vi "Update Status.vi"(8 "error in (no error)":errorcluster, 10 "Value":string, 11 "Status Ref":refnum<vi>) -> (0 "error out":errorcluster)   [LabVIEW 2025, in "I2C Bus Monitor UI.lvlib"]
uses:
  I2C Bus Monitor UI.lvlib
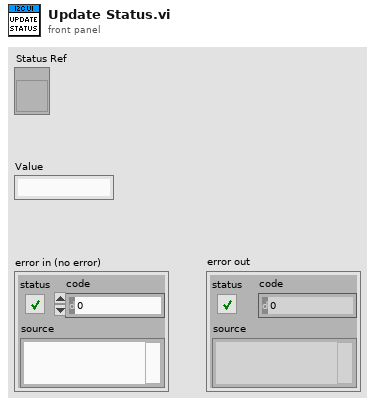
[diagram p1: front panel]
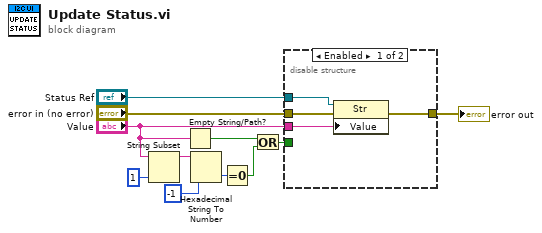
[diagram p0: block diagram]
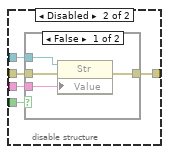
[diagram p2: hidden frame]
diagram:
  n1 = String Subset(string="Value", length (rest)=1 ("length (rest)")) -> (substring=w3:string)  [unwired: 1 in]
  n2 = Empty String/Path?(string/path="Value") -> (empty?=w6:bool)
  n3 = Hexadecimal String To Number(string=w3, default (0uL)=-1 ("default (0 U32)")) -> (number=w7:i32)  [unwired: 1 in, 1 out]
  n4 = Equal To 0?(x=w7) -> (x = 0?=w5:bool)
  n5 = Or(x=w6, y=w5) -> (x .or. y?=w4:bool)
  n6 = disable-structure shown="Enabled" {
    disable-tunnel: [w15 w20] -> w11
    disable-tunnel: "Status Ref" -> [w14 w19]
    disable-tunnel: "error in (no error)" -> [w13 w18]
    disable-tunnel: "Value" -> [w12 w17]
    disable-tunnel: w4 -> [_ w16]
    frame Enabled {
      n7 = property class="Str"(reference=w14, error in=w13, "Value"=w12) -> (error out=w15:errorcluster)  [unwired: 1 out]
    }
    frame Disabled {
      n8 = case shown="False" w16 {
        tunnel: [w24 w25] -> w20
        tunnel: w19 -> [w23 _]
        tunnel: w18 -> [w22 w25]
        tunnel: w17 -> [w21 _]
        frame False {
          n9 = property class="Str"(reference=w23, error in=w22, "Value"=w21) -> (error out=w24:errorcluster)  [unwired: 1 out]
        }
        frame True {
        }
      }
    }
  }
  "error out" <- w11
